vi "Toggle Instrument Display.vi"(8 "error in (no error)":errorcluster, 9 "Instrument":string, 10 "Panel":i32, 11 "Engine in":refnum<class "Engine.lvclass">) -> (0 "error out":errorcluster, 3 "Engine out":refnum<class "Engine.lvclass">)   [LabVIEW 2023, in "Engine.lvlib" / "Engine.lvclass"]
uses:
  Library/Engine.lvclass
  Library/Engine.lvclass/Engine.ctl
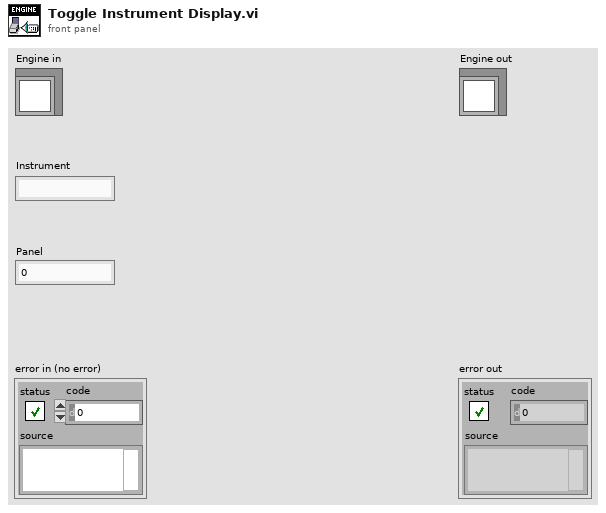
[diagram p1: front panel]
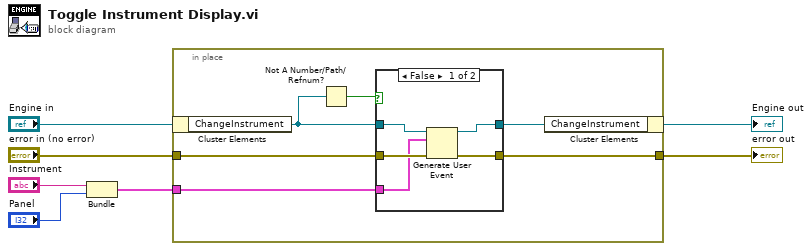
[diagram p0: block diagram]
diagram:
  n1 = Bundle("Instrument"="Instrument", "Panel"="Panel") -> (w1:cluster{"Instrument":string, "Panel":i32})  [unwired: 1 in]
  n2 = in-place {
    in-place-border: "error in (no error)" -> [w10]
    in-place-border: [w9] -> w2
    in-place-border: w1 -> [w8]
    n3 = in-place-cluster #1("Engine in") -> ("ChangeInstrument"=w12:refnum<user-event>)
    n4 = Not A Number/Path/Refnum?(number/path/refnum=w12) -> (NaN/Path/Refnum?=w13:bool)
    n5 = case shown="False" w13 {
      tunnel: w12 -> [w18 w20]
      tunnel: [w17 w20] -> w11
      tunnel: w10 -> [w16 w19]
      tunnel: [w15 w19] -> w9
      tunnel: w8 -> [w14 _]
      frame False {
        n6 = Generate User Event(user event=w18, event data cluster=w14, error in=w16) -> (user event out=w17:refnum<user-event>, error out=w15:errorcluster)  [unwired: 1 in]
      }
      frame True {
      }
    }
    n7 = in-place-cluster #1("ChangeInstrument"=w11) -> (→"Engine out":refnum<class "Engine.lvclass">)
  }
  "error out" <- w2
